vi "Merge get section vim.vi"   [LabVIEW 2020, in "TOML.lvlib"]
uses:
  TOML.lvlib
  54b187fc-e340-4601-a4ea-e075eaf98cce.vi
types:
  T1 = enum16{"open", "replace", "create", "open or create", "replace or create", "replace or create with confirmation"}
  T2 = typedef "TOML.lvlib/TOML Value.ctl" = cluster{"type":enum16{"Table", "Array", "String", "Integer", "Float", "Boolean", "Offset Date-Time", "Local Date-Time", "Local Date", "Local Time", "Path"}, "value":variant}
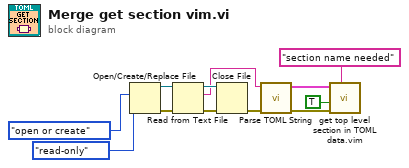
[diagram p0: block diagram]
diagram:
  n1 = Open/Create/Replace File(operation (0:open)=T1."open or create", access (0:read/write)=enum16{"read/write", "read-only", "write-only"}."read-only") -> (refnum out=w8:refnum<file>, error out=w9:errorcluster)  [unwired: 4 in, 1 out]
  n2 = Read from Text File(file (use dialog)=w8, error in=w9) -> (refnum out=w6:refnum<file>, text=w1:string, error out=w7:errorcluster)  [unwired: 2 in, 1 out]
  n3 = Close File(refnum=w6, error in=w7) -> (error out=w4:errorcluster)  [unwired: 1 out]
  n4 = call "Parse TOML String.vi"("error in (no error)"=w4, "String"=w1) -> ("error out"=w2:errorcluster, "Value"=w3:T2)  [unwired: 8 in]
  n5 = call "get top level section in TOML data.vim"("Section name"="section name needed", "error in (no error)"=w2, "Error if missing element"=TRUE, "Value in"=w3) -> ()  [unwired: 5 in, 3 out]
